vi "De-spiked_Stats.vi"(0 "Raw Signal":dbl[](array[numeric]), 1 "No of st dev to chop at":dbl=6.0) -> (2 "mean":dbl format="%.5f", 3 "standard deviation":dbl format="%.5f", 4 "variance":dbl format="%.4f")   [LabVIEW 2022 SP3]
uses:
  <vilib>/Analysis/NI_AALBase.lvlib
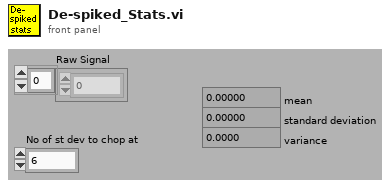
[diagram p1: front panel]
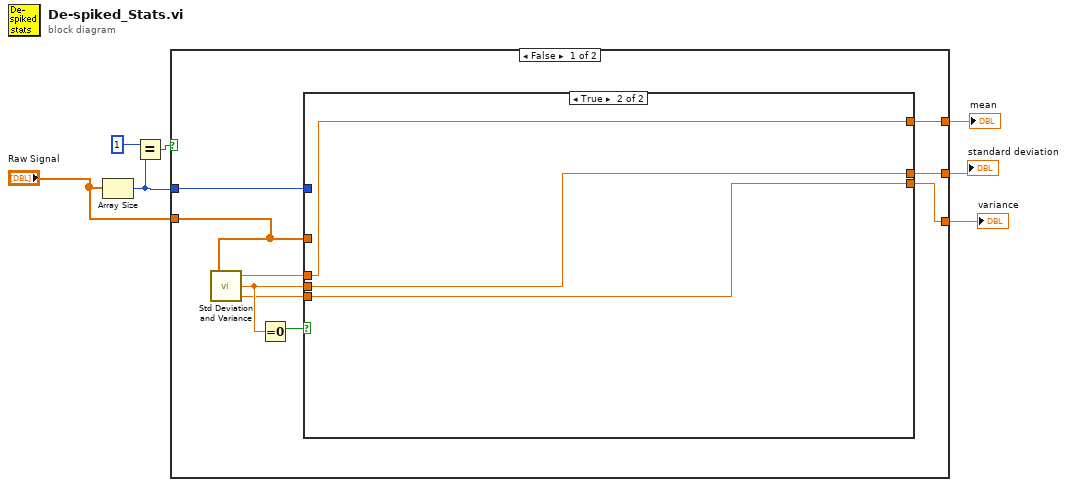
[diagram p0: block diagram]
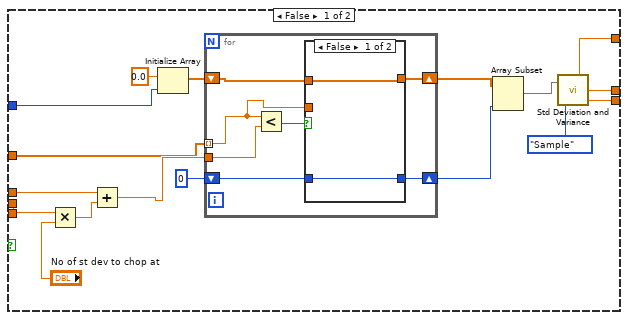
[diagram p2: hidden frame]
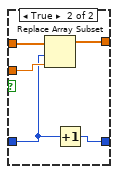
[diagram p3: hidden frame]
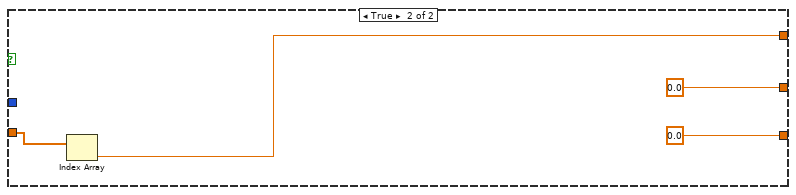
[diagram p4: hidden frame]
diagram:
  n1 = Array Size(array="Raw Signal") -> (size(s)=w3:i32)
  n2 = Equal?(x=1, y=w3) -> (x = y?=w2:bool)
  n3 = case shown="False" w2 {
    tunnel: w3 -> [w16 _]
    tunnel: "Raw Signal" -> [w14 w54]
    tunnel: [w13 w53] -> w6
    tunnel: [w12 0.0 ("standard deviation")] -> w5
    tunnel: [w11 0.0 ("variance")] -> w4
    frame False {
      n4 = call <vilib>:"Std Deviation and Variance.vi"("X"=w14) -> ("mean"=w15:dbl, "standard deviation"=w10:dbl, "variance"=w8:dbl)  [unwired: 1 in]
      n5 = Equal To 0?(x=w10) -> (x = 0?=w9:bool)
      n6 = case shown="True" w9 {
        tunnel: w16 -> [w33 _]
        tunnel: w15 -> [w29 w50]
        tunnel: w10 -> [w28 w49]
        tunnel: w14 -> [w23 _]
        tunnel: [w20 w50] -> w13
        tunnel: [w19 w49] -> w12
        tunnel: [w18 w48] -> w11
        tunnel: w8 -> [_ w48]
        frame False {
          n7 = Multiply(x=w28, y="No of st dev to chop at") -> (x*y=w27:dbl)
          n8 = Add(x=w29, y=w27) -> (x+y=w26:dbl)
          n9 = Initialize Array(0.0 ("element"), w33) -> (w31:dbl[])
          n10 = for {
            shift-right: [w39] -> w25
            shift-left: w31 -> [w40]
            shift-right: [w34] -> w24
            shift-left: 0 -> [w35]
            tunnel: w26 -> [w38]
            tunnel: w23 -> [w36] mode=indexing
            n11 = Less?(x=w36, y=w38) -> (x < y?=w37:bool)
            n12 = case shown="False" w37 {
              tunnel: w40 -> [w41 w47]
              tunnel: [w41 w46] -> w39
              tunnel: w36 -> [_ w45]
              tunnel: w35 -> [w42 w44]
              tunnel: [w42 w43] -> w34
              frame False {
              }
              frame True {
                n13 = Replace Array Subset(array=w47, new element=w45, index=w44) -> (w46:dbl[])
                n14 = Increment(x=w44) -> (x+1=w43:i32)
              }
            }
          }
          n15 = Array Subset(array=w25, length=w24) -> (w22:dbl[])  [unwired: 1 in]
          n16 = call <vilib>:"Std Deviation and Variance.vi"("X"=w22, "Weighting (Sample)"=enum16{"Sample", "Population"}."Sample") -> ("mean"=w20:dbl, "standard deviation"=w19:dbl, "variance"=w18:dbl)
        }
        frame True {
        }
      }
    }
    frame True {
      n17 = Index Array(array=w54) -> (element=w53:dbl)  [unwired: 1 in]
    }
  }
  "mean" <- w6
  "standard deviation" <- w5
  "variance" <- w4
